vi "Lab2_batsound(Ver2).vi"() -> ()   [LabVIEW 2010]
uses:
  <vilib>/sound2/lvsound2.llb/Sound File Read Open.vi
  <vilib>/sound2/lvsound2.llb/Sound File Read (DBL).vi
  <vilib>/measure/maspectr.llb/FFT Spectrum (Mag-Phase) for N Chan.vi
  <vilib>/measure/NI_MAPro.lvlib
panel:
  out "bat  filtered (frequency)":cluster{"f0":dbl, "df":dbl, "magnitude":dbl[]}[](graph)
  out "bat filtered (time)":dynamicdata(graph)
  out "bat (time)":waveform(dbl)[](graph)
  out "bat (frequency)":cluster{"f0":dbl, "df":dbl, "magnitude":dbl[]}[](graph)
  in  "Path":path
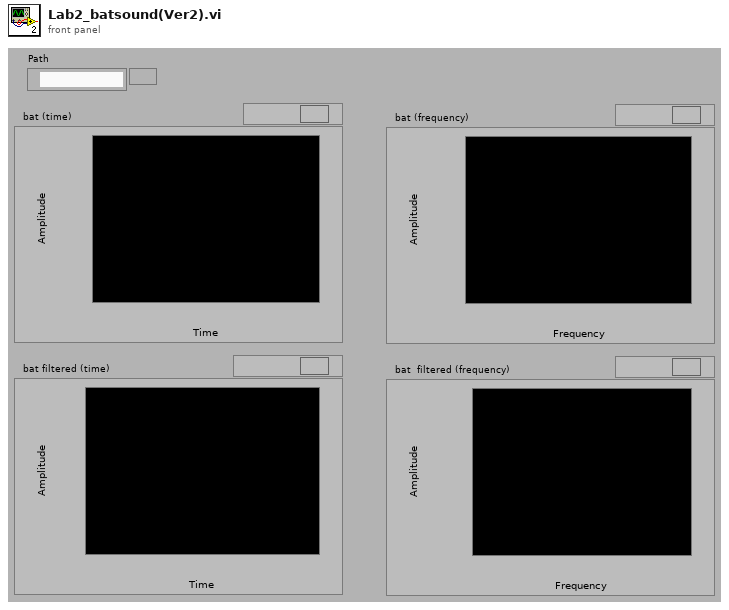
[diagram p1: front panel]
types:
  T1 = typedef "Sound File Refnum.ctl" = refnum<file>
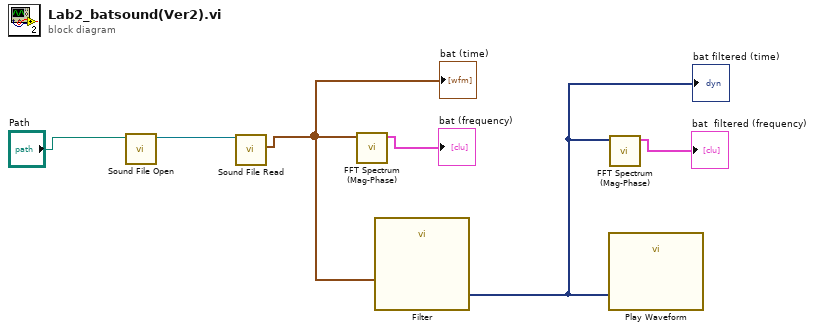
[diagram p0: block diagram]
diagram:
  n1 = call-poly <vilib>:"Sound File Open.vi"("path"="Path") -> ("sound file refnum"=w5:T1)  [unwired: 9 in, 1 out]
  n2 = call-poly <vilib>:"Sound File Read.vi"("sound file refnum"=w5) -> ("data"=w3:waveform(dbl)[])  [unwired: 6 in, 4 out]
  "bat (time)" <- w3
  n3 = call-poly <vilib>:"FFT Spectrum (Mag-Phase).vi"("time signals"=w3) -> ("magnitudes"=→"bat (frequency)":cluster{"f0":dbl, "df":dbl, "magnitude":dbl[]}[])  [unwired: 6 in, 4 out]
  n4 = call "Filter"("Signal"=w3) -> ("Filtered Signal"=w1:dynamicdata)  [unwired: 9 in, 1 out]
  "bat filtered (time)" <- w1
  n5 = call "Play Waveform"("Data"=w1) -> ()  [unwired: 18 in, 1 out]
  n6 = call-poly <vilib>:"FFT Spectrum (Mag-Phase).vi"("time signals"=w1) -> ("magnitudes"=→"bat  filtered (frequency)":cluster{"f0":dbl, "df":dbl, "magnitude":dbl[]}[])  [unwired: 6 in, 4 out]
